vi "Schakelaars.vi"() -> ()   [LabVIEW 2018]
panel:
  in  "stop 2":bool
  in  "digital out":bool[](array[boolean])
  out "Som":dbl
  out "x > y?":bool
  out "Getal":dbl
  in  "stop":bool
  out "analog in":dbl[](array[numeric]) format="%0.2f"
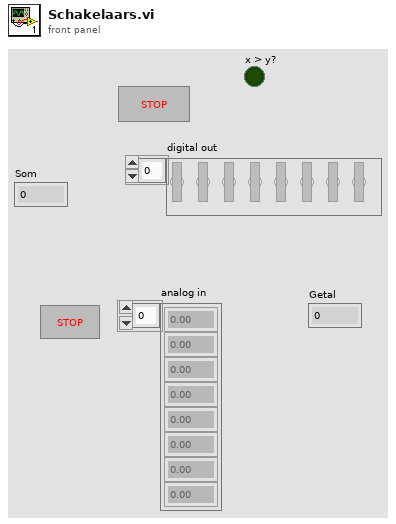
[diagram p1: front panel]
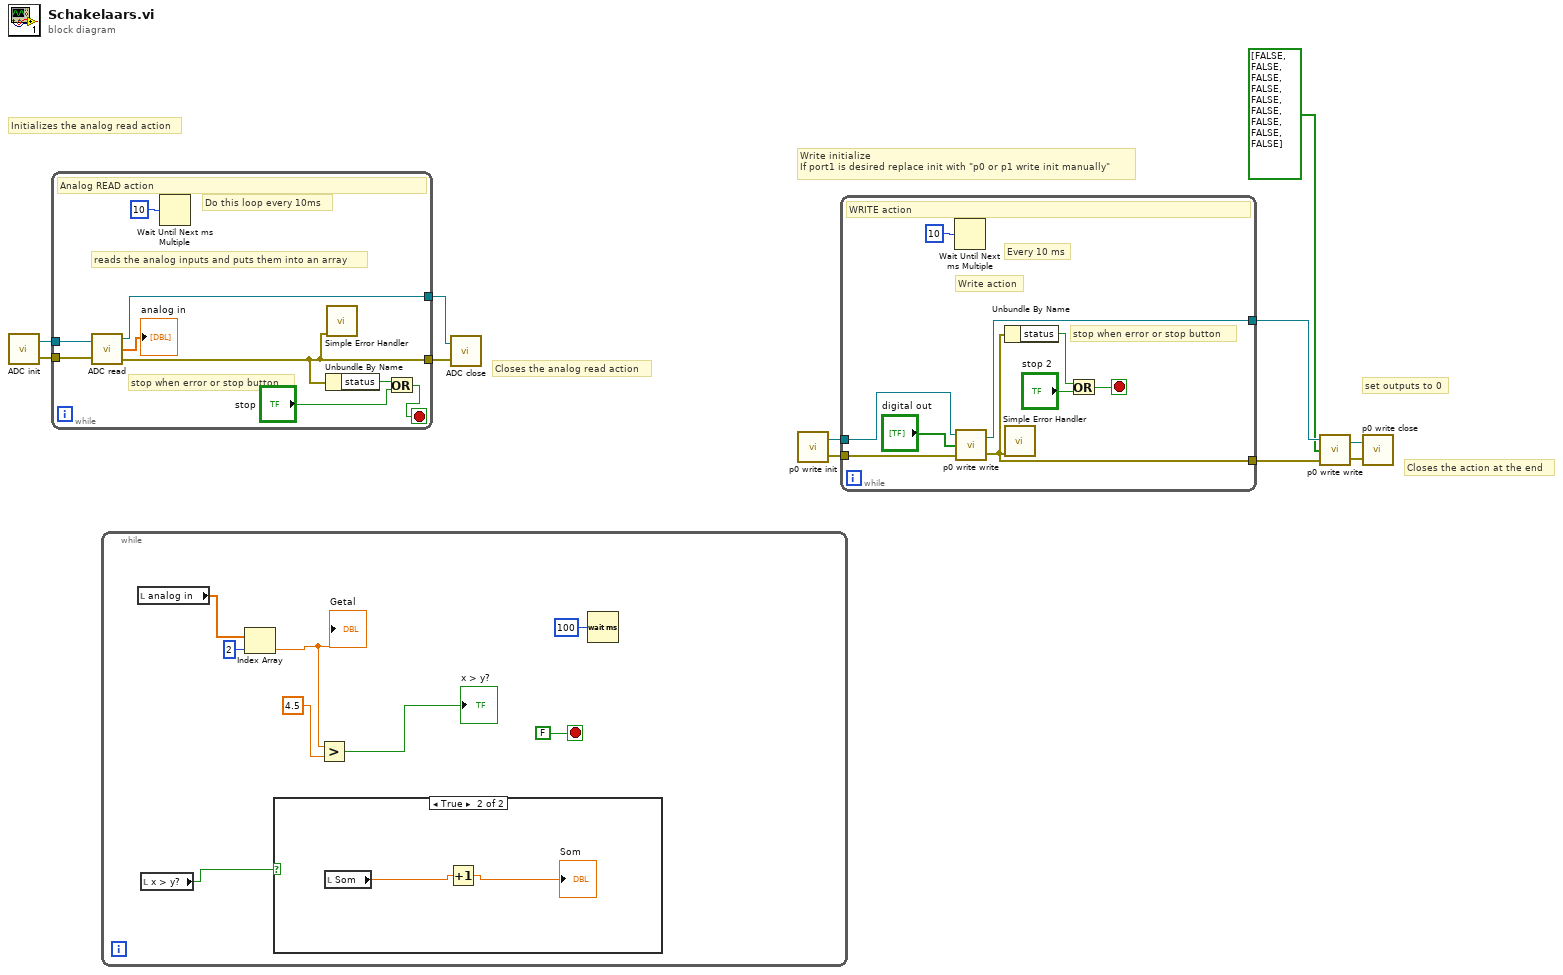
[diagram p0: block diagram]
diagram:
  # "set outputs to 0"
  # "Closes the action at the end"
  # "Write initialize\nIf port1 is desired replace init with \"p0 or p1 write init manually\""
  # "Closes the analog read action"
  # "Initializes the analog read action"
  n1 = call "ADC init.vi"() -> ("error out"=w10:errorcluster, "task out"=w11:refnum<k21>)
  n2 = while {
    tunnel: w11 -> [w20]
    tunnel: w10 -> [w19]
    tunnel: [w15] -> w9
    tunnel: [w18] -> w8
    stop <- w12 stop-if-true
    # "stop when error or stop button"
    # "Do this loop every 10ms"
    # "reads the analog inputs and puts them into an array"
    # "Analog READ action"
    n3 = call "ADC read.vi"("task/channels in"=w20, "error in"=w19) -> ("task out"=w18:refnum<k21>, "analog in"=→"analog in":dbl[], "error out"=w15:errorcluster)
    n4 = Wait Until Next ms Multiple(millisecond multiple=u32 10) -> ()  [unwired: 1 out]
    n5 = Unbundle By Name(w15) -> ("status"=w14:bool)
    n6 = call <vilib>:"Simple Error Handler.vi"("error in (no error)"=w15) -> ()  [unwired: 4 in, 5 out]
    n7 = Or(x=w14, y="stop") -> (x .or. y?=w12:bool)
  }
  n8 = while {
    stop <- FALSE stop-if-true
    n9 = local read "analog in"() -> (w28:dbl[])
    n10 = local read "x > y?"() -> (w25:bool)
    n11 = Index Array(array=w28, index=2) -> (element=w22:dbl)
    "Getal" <- w22
    n12 = case shown="True" w25 {
      frame False {
      }
      frame True {
        n13 = local read "Som"() -> (w30:dbl)
        n14 = Increment(x=w30) -> (x+1=→"Som":dbl)
      }
    }
    n15 = Greater?(x=w22, y=4.5) -> (0:→"x > y?":bool)
    n16 = Wait (ms)(milliseconds to wait=u32 100) -> ()  [unwired: 1 out]
  }
  n17 = call "ADC close.vi"("error in"=w9, "task/channels in"=w8) -> ()
  n18 = call "p0 write init.vi"() -> ("error out"=w2:errorcluster, "task out"=w3:refnum<k21>)
  n19 = while {
    tunnel: w3 -> [w39]
    tunnel: [w38] -> w7
    tunnel: w2 -> [w37]
    tunnel: [w32] -> w6
    stop <- w33 stop-if-true
    # "stop when error or stop button"
    # "Every 10 ms"
    # "Write action"
    # "WRITE action"
    n20 = Wait Until Next ms Multiple(millisecond multiple=u32 10) -> ()  [unwired: 1 out]
    n21 = call "p0 write write.vi"("error in"=w37, "digital out"="digital out", "task/channels in"=w39) -> ("error out"=w32:errorcluster, "task out"=w38:refnum<k21>)
    n22 = Unbundle By Name(w32) -> ("status"=w31:bool)
    n23 = call <vilib>:"Simple Error Handler.vi"("error in (no error)"=w32) -> ()  [unwired: 4 in, 5 out]
    n24 = Or(x=w31, y="stop 2") -> (x .or. y?=w33:bool)
  }
  n25 = call "p0 write write.vi"("error in"=w6, "digital out"=bool[] [FALSE, FALSE, FALSE, FALSE, FALSE, FALSE, FALSE, FALSE, FALSE], "task/channels in"=w7) -> ("error out"=w4:errorcluster, "task out"=w5:refnum<k21>)
  n26 = call "p0 write close.vi"("error in"=w4, "task/channels in"=w5) -> ()
